vi "3_cubic_sum(170382,170307).vi"() -> ()   [LabVIEW 2015]
panel:
  out "x+y":i64
  in  "final value":i64
  in  "initial value":i64
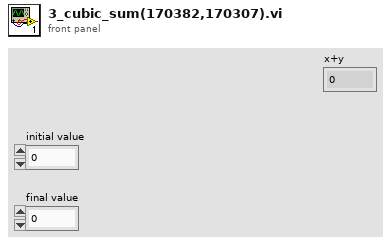
[diagram p1: front panel]
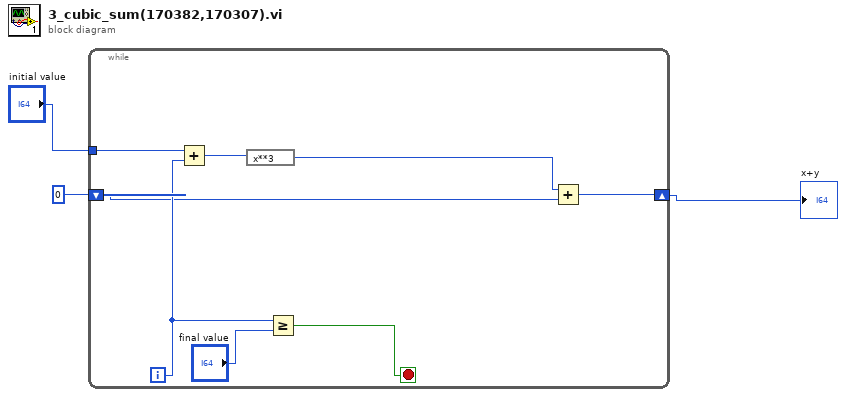
[diagram p0: block diagram]
diagram:
  n1 = while {
    shift-right: [w4] -> w1
    shift-left: i64 0 -> [w5]
    tunnel: "initial value" -> [w7]
    i -> [w8]
    stop <- w10 stop-if-true
    n2 = Add(x=w7, y=w8) -> (x+y=w9:i64)
    n3 = expression code="x**3"(w9) -> (w6:i64)
    n4 = Greater Or Equal?(x=w8, y="final value") -> (x >= y?=w10:bool)
    n5 = Add(x=w6, y=w5) -> (x+y=w4:i64)
  }
  "x+y" <- w1
